vi "Validate RaF Custom Device Configuration.vi"(8 "error in (no error)":errorcluster, 11 "Routing and Faulting Custom Device Ref in":T1 format="%.0x") -> (0 "error out":errorcluster, 3 "Routing and Faulting Custom Device Ref out":T1 format="%.0x")   [LabVIEW 2017, in "Routing and Faulting Scripting.lvlib"]
uses:
  Routing and Faulting Scripting.lvlib
  <vilib>/NI Veristand/Custom Device API/Custom Device Item Ref.ctl
  <vilib>/NI Veristand/Custom Device API/Custom Device API.lvlib
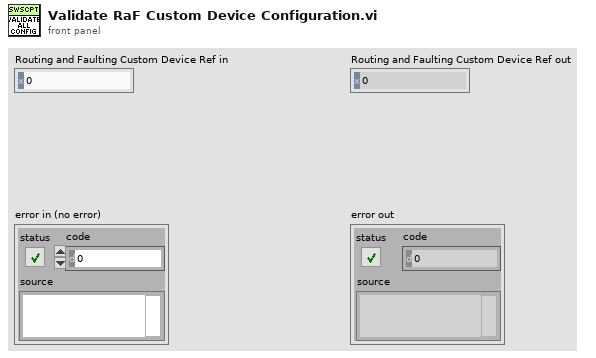
[diagram p1: front panel]
types:
  T1 = typedef "Custom Device API.lvlib/Custom Device Item Ref.ctl" = u64
  T2 = typedef "Routing and Faulting Scripting.lvlib/Module Connection Information.ctl" = cluster{"Module Path":string, "Model":string, "Possible Connections":T3[]}
  T3 = typedef "Routing and Faulting Hardware API.lvlib/Possible Connections for Endpoint.ctl" = cluster{"Source":string, "Destinations":string[]}
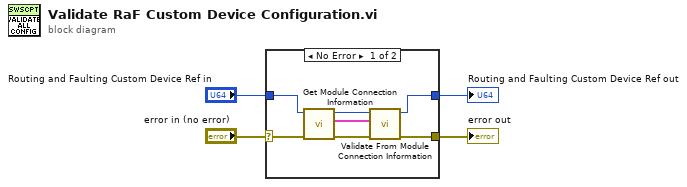
[diagram p0: block diagram]
diagram:
  n1 = case shown="No Error" "error in (no error)" {
    selector: "error in (no error)" -> [w5 w13]
    tunnel: [w8 w13] -> w4
    tunnel: "Routing and Faulting Custom Device Ref in" -> [w7 w12]
    tunnel: [w6 w12] -> w2
    frame No Error {
      n2 = call "Get Module Connection Information.vi"("error in (no error)"=w5, "Routing and Faulting Custom Device Ref in"=w7) -> ("error out"=w11:errorcluster, "Module Connection Information"=w10:T2[], "Routing and Faulting Custom Device Ref out"=w9:T1)  [unwired: 7 in]
      n3 = call "Validate From Module Connection Information.vi"("error in (no error)"=w11, "Module Connection Information"=w10, "Routing and Faulting Custom Device Ref in"=w9) -> ("error out"=w8:errorcluster, "Routing and Faulting Custom Device Ref out"=w6:T1)  [unwired: 7 in]
    }
    frame Error {
    }
  }
  "Routing and Faulting Custom Device Ref out" <- w2
  "error out" <- w4
